vi "Pre Launch Init.vi"(11 "Nested in":refnum<class "ACQ Contador.lvclass">) -> (0 "error out":errorcluster, 3 "Nested out":refnum<class "ACQ Contador.lvclass">)   [LabVIEW 2020, in "ACQ Contador.lvlib" / "ACQ Contador.lvclass"]
doc: "(<B>Filename</B>: Actor Framework.lvlib:Actor.lvclass:Pre Launch Init.vi)\n\nDefines behavior that occurs after the Launch Nested Actor method is invoked but before the actor's Actor Core method begins running.\n\nBy default, this method does nothing. A descendant class may override it to define behavior."
uses:
  ACQ Contador.lvclass
  ACQ Contador.lvclass/ACQ Contador.ctl
  <vilib>/ActorFramework/Actor/Actor.lvclass
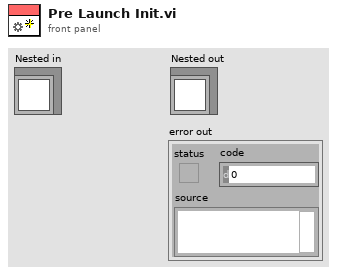
[diagram p1: front panel]
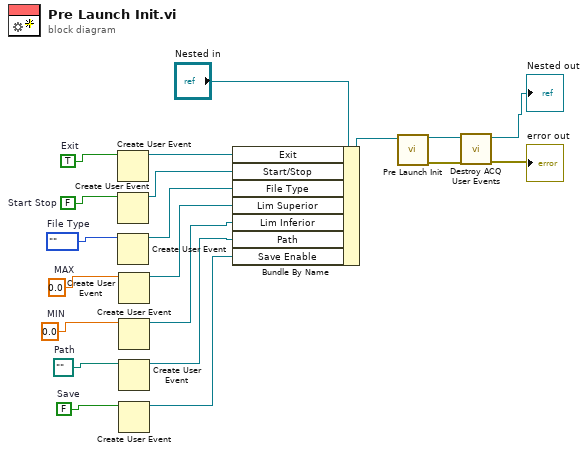
[diagram p0: block diagram]
diagram:
  w5 = path ""  # Path
  w6 = 0.0  # MIN
  w7 = 0.0  # MAX
  w8 = enum16{""}.""  # File Type
  w9 = FALSE  # Save
  w10 = FALSE  # Start Stop
  w11 = TRUE  # Exit
  n1 = Create User Event(user event datatype=w11) -> (user event=w18:refnum<user-event>)  [unwired: 1 in, 1 out]
  n2 = Create User Event(user event datatype=w10) -> (user event=w17:refnum<user-event>)  [unwired: 1 in, 1 out]
  n3 = Create User Event(user event datatype=w8) -> (user event=w16:refnum<user-event>)  [unwired: 1 in, 1 out]
  n4 = Create User Event(user event datatype=w7) -> (user event=w15:refnum<user-event>)  [unwired: 1 in, 1 out]
  n5 = Create User Event(user event datatype=w6) -> (user event=w14:refnum<user-event>)  [unwired: 1 in, 1 out]
  n6 = Create User Event(user event datatype=w5) -> (user event=w13:refnum<user-event>)  [unwired: 1 in, 1 out]
  n7 = Create User Event(user event datatype=w9) -> (user event=w12:refnum<user-event>)  [unwired: 1 in, 1 out]
  n8 = Bundle By Name(cluster="Nested in", "Exit"=w18, "Start/Stop"=w17, "File Type"=w16, "Lim Superior"=w15, "Lim Inferior"=w14, "Path"=w13, "Save Enable"=w12) -> (w19:refnum<class "ACQ Contador.lvclass">)
  n9 = call-parent "Pre Launch Init.vi"("Actor in"=w19) -> ("error out"=w4:errorcluster, "Actor out"=w1:refnum<class "ACQ Contador.lvclass">)  [unwired: 9 in]
  n10 = call "Destroy ACQ User Events.vi"("error in (no error)"=w4, "ACQ Contador in"=w1) -> ("error out"=→"error out":errorcluster, "ACQ Contador out"=→"Nested out":refnum<class "ACQ Contador.lvclass">)  [unwired: 8 in]
